vi "Pre Launch Init.vi"(11 "Nested in":refnum<class "Message Actor.lvclass">) -> (0 "error out":errorcluster, 3 "Nested out":refnum<class "Message Actor.lvclass">)   [LabVIEW 2020, in "Message Actor.lvlib" / "Message Actor.lvclass"]
doc: "(<B>Filename</B>: Actor Framework.lvlib:Actor.lvclass:Pre Launch Init.vi)\n\nDefines behavior that occurs after the Launch Nested Actor method is invoked but before the actor's Actor Core method begins running.\n\nBy default, this method does nothing. A descendant class may override it to define behavior."
uses:
  Message Actor.lvclass
  Message Actor.lvclass/Message Actor.ctl
  SubPanel Actor/SubPanel Actor/SubPanel Actor.lvclass
  Message Actor Messages/Send Message Msg/Send Message Msg.lvclass
  <vilib>/ActorFramework/Actor/Actor.lvclass
  C:/Users/eddiews/Documents/Git Hub Repositorios/VendingMachine_ActorFramework/SubPanel Actor/SubPanel Actor/SubPanel Actor.lvclass
  C:/Program Files (x86)/National Instruments/LabVIEW 2020/vi.lib/ActorFramework/Actor/Actor.lvclass
  C:/Users/eddiews/Documents/Git Hub Repositorios/VendingMachine_ActorFramework/Message Actor/Message Actor.lvclass
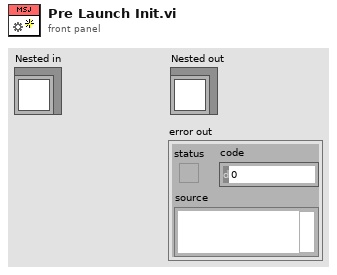
[diagram p1: front panel]
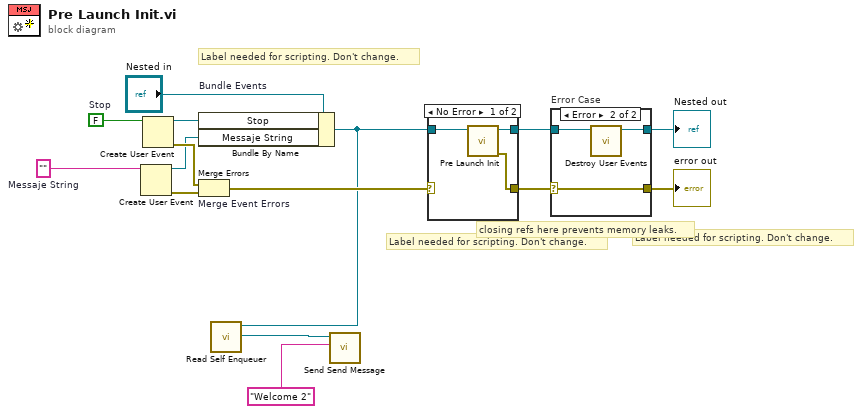
[diagram p0: block diagram]
diagram:
  w6 = ""  # Messaje String
  w14 = FALSE  # Stop
  # "Label needed for scripting. Don't change."
  # "Label needed for scripting. Don't change."
  # "Label needed for scripting. Don't change."
  # "closing refs here prevents memory leaks."
  n1 = Create User Event(user event datatype=w6) -> (user event=w5:refnum<user-event>, error out=w4:errorcluster)  [unwired: 1 in]
  n2 = Create User Event(user event datatype=w14) -> (user event=w11:refnum<user-event>, error out=w13:errorcluster)  [unwired: 1 in]
  n3 = Bundle By Name "Bundle Events"(cluster="Nested in", "Stop"=w11, "Messaje String"=w5) -> (w1:refnum<class "Message Actor.lvclass">)
  n4 = Merge Errors "Merge Event Errors"(w13, w4) -> (w8:errorcluster)
  n5 = call <vilib>:"Read Self Enqueuer.vi"("Actor"=w1) -> ("Self Enqueuer"=w3:refnum<class "Message Enqueuer.lvclass">)  [unwired: 10 in]
  n6 = call "Send Send Message.vi"("Messaje"="Welcome 2", "Message Enqueuer"=w3) -> ()  [unwired: 8 in, 2 out]
  n7 = case shown="No Error" w8 {
    selector: w8 -> [_ w20]
    tunnel: [w18 w19] -> w9
    tunnel: w1 -> [w17 w19]
    tunnel: [w16 w20] -> w7
    frame No Error {
      n8 = call-parent "Pre Launch Init.vi"("SubPanel Actor in"=w17) -> ("error out"=w16:errorcluster, "SubPanel Actor out"=w18:refnum<class "Message Actor.lvclass">)  [unwired: 9 in]
    }
    frame Error {
    }
  }
  n9 = case "Error Case" shown="Error" w7 {
    selector: w7 -> [w21 w25]
    tunnel: w9 -> [w22 w24]
    tunnel: [w22 w23] -> w12
    tunnel: [w21 w25] -> w10
    frame No Error {
    }
    frame Error {
      n10 = call "Destroy User Events.vi"("UI Template in"=w24) -> ("UI Template out"=w23:refnum<class "Message Actor.lvclass">)  [unwired: 10 in]
    }
  }
  "error out" <- w10
  "Nested out" <- w12
